vi "attachments.get.vi"(8 "error in (no error)":errorcluster, 11 "Run in":refnum<class "Run.lvclass">) -> (0 "error out":errorcluster, 2 "attachments":string[](array[string]), 3 "Run out":refnum<class "Run.lvclass">)   [LabVIEW 2020, in "Run.lvclass"]
uses:
  Run.lvclass
  Run.lvclass/Run.ctl
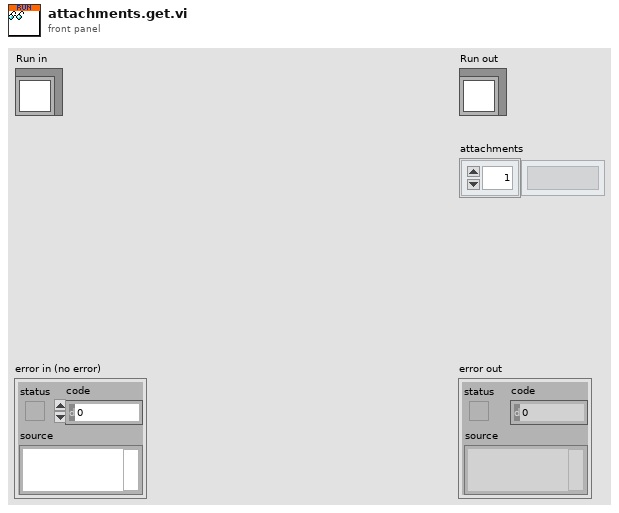
[diagram p1: front panel]
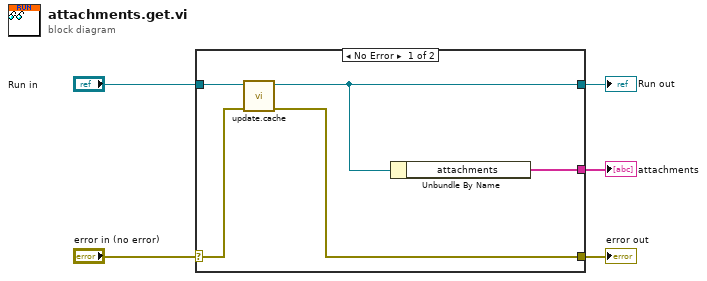
[diagram p0: block diagram]
diagram:
  n1 = case shown="No Error" "error in (no error)" {
    selector: "error in (no error)" -> [w10 w11]
    tunnel: [w8 w11] -> w4
    tunnel: [w6 w12] -> w2
    tunnel: "Run in" -> [w7 w12]
    tunnel: [w9 _] -> w1
    frame No Error {
      n2 = call "update.cache.vi"("error in"=w10, "Run in"=w7) -> ("error out"=w8:errorcluster, "Run out"=w6:refnum<class "Run.lvclass">)  [unwired: 8 in]
      n3 = Unbundle By Name(w6) -> ("attachments"=w9:string[])
    }
    frame Error {
    }
  }
  "error out" <- w4
  "Run out" <- w2
  "attachments" <- w1
